vi "HFP Generator.vi"() -> ()   [LabVIEW 2015]
doc: "Example VI that demonstrates all library features."
uses:
  PL HFP Generator.lvclass
panel:
  in  "series":u16(ring) items=["Plasma G20", "Plasma GK"]
  in  "read configuration":bool
  out "measurements":T1 {"SWR timer state" items=["off"=0, "counting"=2, "counting and skipping"=3, "protection"=4]; "rf power"."Ppump, W" items=["500", "1000", "2000", "3000", "4000", "6000", "8000"]; "power ramp state" items=["off", "ramp up", "full power", "ramp down", "off, awaiting reset"]}
  in  "configuration":T2={"power on"=FALSE, "rf on"=FALSE, "control mode"=0, "disable rf"=FALSE, "power"={"Pfwd, W"=50, "Pload, W"=50, "Pmax, W"=1000, "ramp"={"mode"=0, "up time, s"=0, "down time, s"=0}}, "modulation"={"mode"=0, "f, Hz"=1000, "pulse time, s"=1.0, "duty cycle, %"=50.0, "Ppause, W"=50}, "SWR timer"={"on"=FALSE, "Pthreshold, W"=0, "count time, s"=0, "skip time, s"=0}, "phase"={"phase, °"=0.0, "mode"=1}} {"phase"."mode" items=["slave", "master"]; "modulation"."mode" items=["off"=0, "internal full"=2, "internal partial"=3, "external full"=4, "external partial"=5]; "power"."ramp"."mode" items=["off", "ramp up", "ramp up and down", "ramp down"]; "control mode" items=["Pload", "Pfwd"]}
  out "device information":T3
  in  "stop bits":u16(ring)=10 items=["1.0"=10, "2.0"=20]
  in  "parity":enum16{"None", "Odd", "Even", "Mark", "Space"}(ring)
  out "HFP Gen":refnum<class "PL HFP Generator.lvclass">
  in  "port":refnum<visa-resource-name>
  in  "address":u8=1
  in  "baud rate":u32(ring)=19200 items=["9600"=9600, "19200"=19200, "38400"=38400]
  out "error":errorcluster
  in  "stop":bool
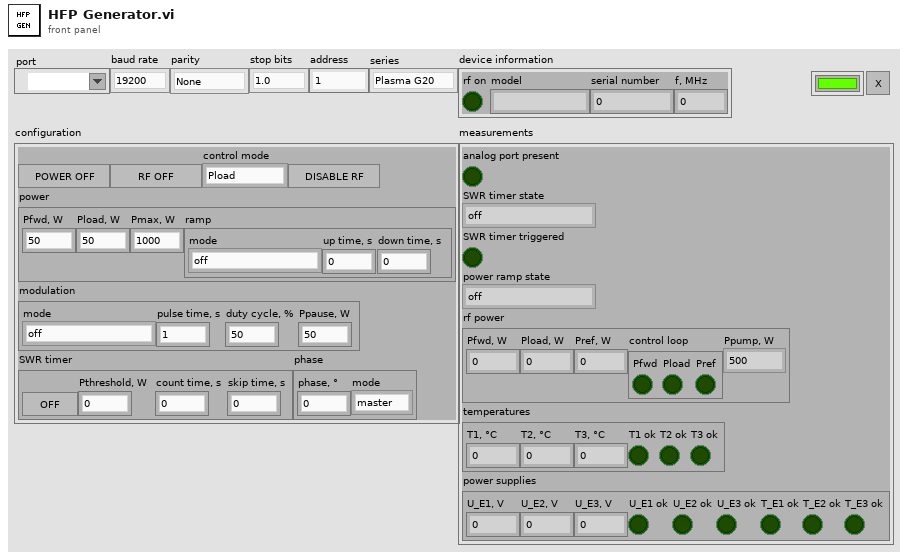
[diagram p1: front panel]
types:
  T1 = cluster{"analog port present":bool, "SWR timer state":u8, "SWR timer triggered":bool, "power ramp state":u8, "rf power":cluster{"Pfwd, W":dbl, "Pload, W":dbl, "Pref, W":dbl, "control loop":cluster{"Pfwd":bool, "Pload":bool, "Pref":bool}, "Ppump, W":u8}, "temperatures":cluster{"T1, °C":dbl, "T2, °C":dbl, "T3, °C":dbl, "T1 ok":bool, "T2 ok":bool, "T3 ok":bool}, "power supplies":cluster{"U_E1, V":dbl, "U_E2, V":dbl, "U_E3, V":dbl, "U_E1 ok":bool, "U_E2 ok":bool, "U_E3 ok":bool, "T_E1 ok":bool, "T_E2 ok":bool, "T_E3 ok":bool}}
  T2 = cluster{"power on":bool, "rf on":bool, "control mode":u8, "disable rf":bool, "power":cluster{"Pfwd, W":u16, "Pload, W":u16, "Pmax, W":u16, "ramp":cluster{"mode":u8, "up time, s":u8, "down time, s":u8}}, "modulation":cluster{"mode":u8, "f, Hz":u16, "pulse time, s":dbl, "duty cycle, %":dbl, "Ppause, W":u16}, "SWR timer":cluster{"on":bool, "Pthreshold, W":u8, "count time, s":u8, "skip time, s":u8}, "phase":cluster{"phase, °":dbl, "mode":u8}}
  T3 = cluster{"rf on":bool, "model":string, "serial number":u16, "f, MHz":dbl}
  T4 = cluster{"power on":bool, "rf on":bool, "control mode":u8, "modulation mode":u8, "SWR timer on":bool, "power ramp mode":u8}
  T5 = cluster{"power on":bool, "rf on":bool, "control mode":u8, "mode":u8, "on":bool, "disable rf":bool}
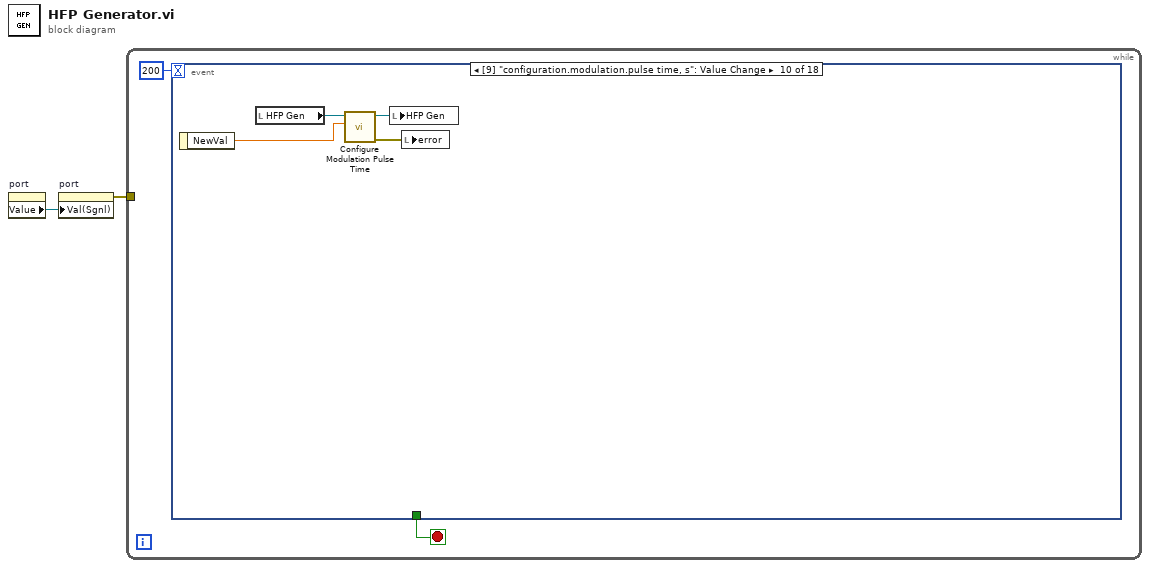
[diagram p0: block diagram]
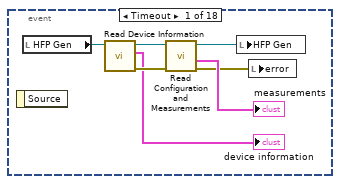
[diagram p2: hidden frame]
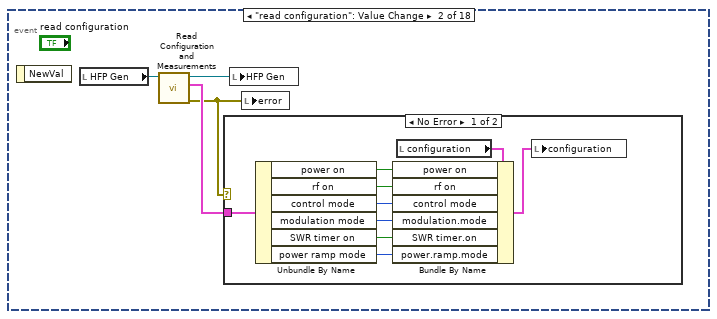
[diagram p3: hidden frame]
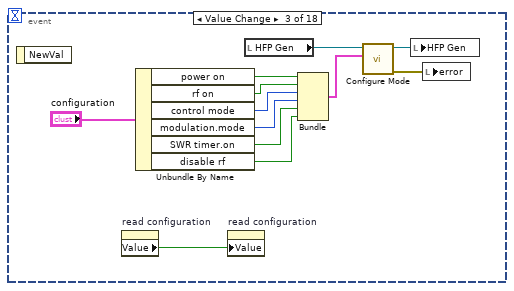
[diagram p5: hidden frame]
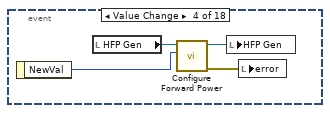
[diagram p6: hidden frame]
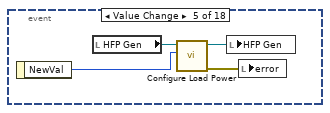
[diagram p7: hidden frame]
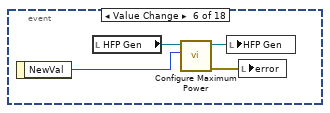
[diagram p8: hidden frame]
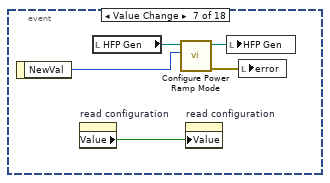
[diagram p9: hidden frame]
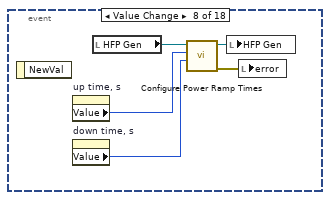
[diagram p10: hidden frame]
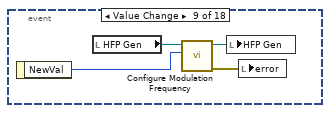
[diagram p11: hidden frame]
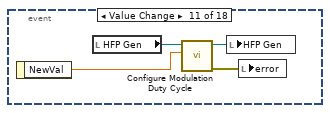
[diagram p12: hidden frame]
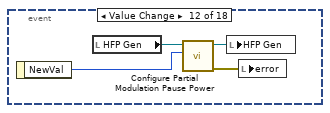
[diagram p13: hidden frame]
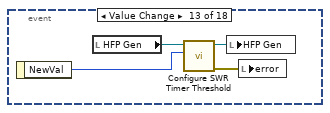
[diagram p14: hidden frame]
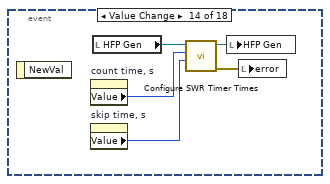
[diagram p15: hidden frame]
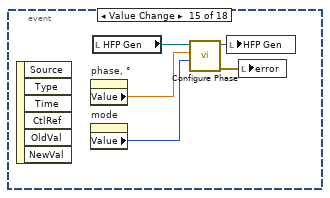
[diagram p16: hidden frame]
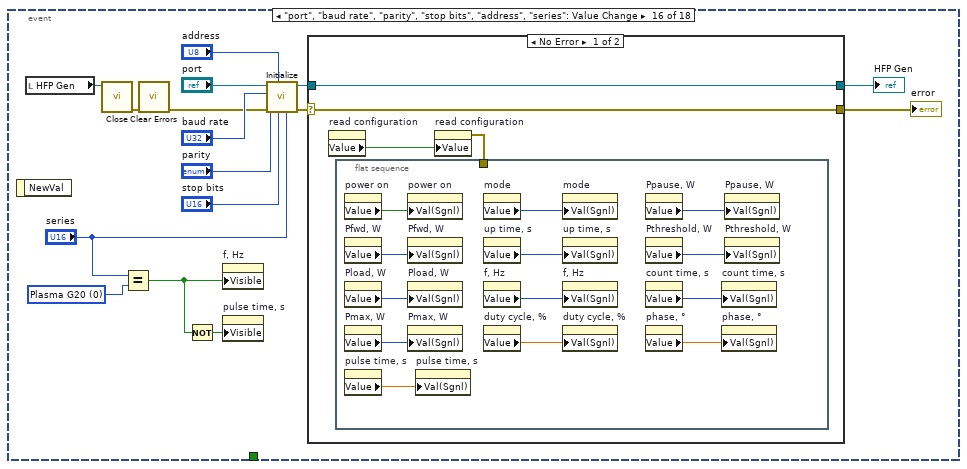
[diagram p17: hidden frame]
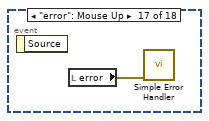
[diagram p19: hidden frame]
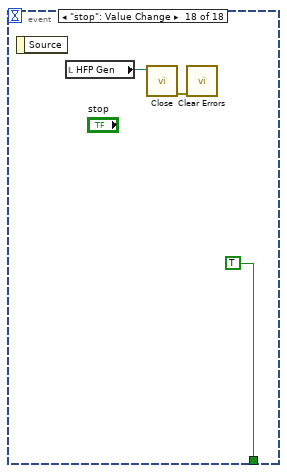
[diagram p20: hidden frame]
diagram:
  n1 = property on="port" class="VISAName"() -> ("Value"=w1:refnum<visa-resource-name>)  [unwired: 2 in, 2 out]
  n2 = property on="port" class="VISAName"("Val(Sgnl)"=w1) -> (error out=w2:errorcluster)  [unwired: 2 in, 1 out]
  n3 = while {
    tunnel: w2 -> [_]
    stop <- w3 stop-if-true
    n4 = event shown="[9] \"configuration.modulation.pulse time, s\": Value Change" {
      selector: _ -> [_ _ _ _ _ _ _ _ _ _ _ _ _ _ _ _ _ _]
      dyn-events: _ -> [_ _ _ _ _ _ _ _ _ _ _ _ _ _ _ _ _ _]
      timeout: 200 -> [_ _ _ _ _ _ _ _ _ _ _ _ _ _ _ _ _ _]
      tunnel: [_ _ _ _ _ _ _ _ _ _ _ _ _ _ _ _ _ TRUE ("stop")] -> w3
      event Timeout {
        n5 = event-data() -> ()  [unwired: 1 in, 1 out]
        n6 = local read "HFP Gen"() -> (w11:refnum<class "PL HFP Generator.lvclass">)
        n7 = call "Read Device Information.vi"("HFP Gen in"=w11) -> ("error out"=w8:errorcluster, "information"=→"device information":T3, "HFP Gen out"=w10:refnum<class "PL HFP Generator.lvclass">)  [unwired: 8 in]
        n8 = call "Read Configuration and Measurements.vi"("error in (no error)"=w8, "HFP Gen in"=w10) -> ("error out"=w5:errorcluster, "measurements"=→"measurements":T1, "HFP Gen out"=w9:refnum<class "PL HFP Generator.lvclass">)  [unwired: 6 in, 1 out]
        n9 = local write "HFP Gen"(w9) -> ()
        n10 = local write "error"(w5) -> ()
      }
      event "read configuration": Value Change {
        n11 = event-data() -> ()  [unwired: 1 in, 1 out]
        n12 = local read "HFP Gen"() -> (w15:refnum<class "PL HFP Generator.lvclass">)
        n13 = call "Read Configuration and Measurements.vi"("HFP Gen in"=w15) -> ("error out"=w12:errorcluster, "configuration"=w13:T4, "HFP Gen out"=w14:refnum<class "PL HFP Generator.lvclass">)  [unwired: 7 in, 1 out]
        n14 = case shown="No Error" w12 {
          tunnel: w13 -> [w24 _]
          frame No Error {
            n15 = Unbundle By Name(w24) -> ("power on"=w22:bool, "rf on"=w21:bool, "control mode"=w20:u8, "modulation mode"=w19:u8, "SWR timer on"=w18:bool, "power ramp mode"=w17:u8)
            n16 = local read "configuration"() -> (w16:T2)
            n17 = Bundle By Name(cluster=w16, "power on"=w22, "rf on"=w21, "control mode"=w20, "modulation.mode"=w19, "SWR timer.on"=w18, "power.ramp.mode"=w17) -> (w23:T2)
            n18 = local write "configuration"(w23) -> ()
          }
          frame Error {
          }
        }
        n19 = local write "HFP Gen"(w14) -> ()
        n20 = local write "error"(w12) -> ()
      }
      event "configuration.power on", "configuration.rf on", "configuration.control mode", "configuration.modulation.mode", "configuration.SWR timer.on", "configuration.disable rf": Value Change {
        n21 = event-data() -> ()  [unwired: 1 in, 1 out]
        n22 = property on="read configuration" class="Bool (strict)"() -> ("Value"=w25:bool)  [unwired: 2 in, 2 out]
        n23 = Unbundle By Name("configuration") -> ("power on"=w32:bool, "rf on"=w31:bool, "control mode"=w30:u8, "modulation.mode"=w29:u8, "SWR timer.on"=w28:bool, "disable rf"=w27:bool)
        n24 = property on="read configuration" class="Bool (strict)"("Value"=w25) -> ()  [unwired: 2 in, 2 out]
        n25 = local read "HFP Gen"() -> (w34:refnum<class "PL HFP Generator.lvclass">)
        n26 = Bundle("power on"=w32, "rf on"=w31, "control mode"=w30, "mode"=w29, "on"=w28, "disable rf"=w27) -> (w26:T5)  [unwired: 1 in]
        n27 = call "Configure Mode.vi"("mode"=w26, "HFP Gen in"=w34) -> ("error out"=w36:errorcluster, "HFP Gen out"=w35:refnum<class "PL HFP Generator.lvclass">)  [unwired: 8 in]
        n28 = local write "HFP Gen"(w35) -> ()
        n29 = local write "error"(w36) -> ()
      }
      event "configuration.power.Pfwd, W": Value Change {
        n30 = event-data() -> ("NewVal"=w37:u16)  [unwired: 1 in]
        n31 = local read "HFP Gen"() -> (w40:refnum<class "PL HFP Generator.lvclass">)
        n32 = call "Configure Forward Power.vi"("Pfwd, W"=w37, "HFP Gen in"=w40) -> ("error out"=w38:errorcluster, "HFP Gen out"=w39:refnum<class "PL HFP Generator.lvclass">)  [unwired: 8 in]
        n33 = local write "HFP Gen"(w39) -> ()
        n34 = local write "error"(w38) -> ()
      }
      event "configuration.power.Pload, W": Value Change {
        n35 = event-data() -> ("NewVal"=w41:u16)  [unwired: 1 in]
        n36 = local read "HFP Gen"() -> (w43:refnum<class "PL HFP Generator.lvclass">)
        n37 = call "Configure Load Power.vi"("Pload, W"=w41, "HFP Gen in"=w43) -> ("error out"=w42:errorcluster, "HFP Gen out"=w44:refnum<class "PL HFP Generator.lvclass">)  [unwired: 8 in]
        n38 = local write "HFP Gen"(w44) -> ()
        n39 = local write "error"(w42) -> ()
      }
      event "configuration.power.Pmax, W": Value Change {
        n40 = event-data() -> ("NewVal"=w45:u16)  [unwired: 1 in]
        n41 = local read "HFP Gen"() -> (w46:refnum<class "PL HFP Generator.lvclass">)
        n42 = call "Configure Maximum Power.vi"("Pmax, W"=w45, "HFP Gen in"=w46) -> ("error out"=w47:errorcluster, "HFP Gen out"=w48:refnum<class "PL HFP Generator.lvclass">)  [unwired: 8 in]
        n43 = local write "HFP Gen"(w48) -> ()
        n44 = local write "error"(w47) -> ()
      }
      event "configuration.power.ramp.mode": Value Change {
        n45 = event-data() -> ("NewVal"=w50:u8)  [unwired: 1 in]
        n46 = property on="read configuration" class="Bool (strict)"() -> ("Value"=w49:bool)  [unwired: 2 in, 2 out]
        n47 = local read "HFP Gen"() -> (w51:refnum<class "PL HFP Generator.lvclass">)
        n48 = call "Configure Power Ramp Mode.vi"("power ramp mode"=w50, "HFP Gen in"=w51) -> ("error out"=w52:errorcluster, "HFP Gen out"=w53:refnum<class "PL HFP Generator.lvclass">)  [unwired: 8 in]
        n49 = property on="read configuration" class="Bool (strict)"("Value"=w49) -> ()  [unwired: 2 in, 2 out]
        n50 = local write "HFP Gen"(w53) -> ()
        n51 = local write "error"(w52) -> ()
      }
      event "configuration.power.ramp.up time, s", "configuration.power.ramp.down time, s": Value Change {
        n52 = event-data() -> ()  [unwired: 1 in, 1 out]
        n53 = property on="up time, s" class="DigNum (strict)"() -> ("Value"=w55:u8)  [unwired: 2 in, 2 out]
        n54 = property on="down time, s" class="DigNum (strict)"() -> ("Value"=w54:u8)  [unwired: 2 in, 2 out]
        n55 = local read "HFP Gen"() -> (w56:refnum<class "PL HFP Generator.lvclass">)
        n56 = call "Configure Power Ramp Times.vi"("ramp-down time, s"=w54, "ramp-up time, s"=w55, "HFP Gen in"=w56) -> ("error out"=w57:errorcluster, "HFP Gen out"=w58:refnum<class "PL HFP Generator.lvclass">)  [unwired: 7 in]
        n57 = local write "HFP Gen"(w58) -> ()
        n58 = local write "error"(w57) -> ()
      }
      event "configuration.modulation.f, Hz": Value Change {
        n59 = event-data() -> ("NewVal"=w59:u16)  [unwired: 1 in]
        n60 = local read "HFP Gen"() -> (w61:refnum<class "PL HFP Generator.lvclass">)
        n61 = call "Configure Modulation Frequency.vi"("f, Hz"=w59, "HFP Gen in"=w61) -> ("error out"=w60:errorcluster, "HFP Gen out"=w62:refnum<class "PL HFP Generator.lvclass">)  [unwired: 8 in]
        n62 = local write "HFP Gen"(w62) -> ()
        n63 = local write "error"(w60) -> ()
      }
      event "configuration.modulation.pulse time, s": Value Change {
        n64 = event-data() -> ("NewVal"=w63:dbl)  [unwired: 1 in]
        n65 = local read "HFP Gen"() -> (w65:refnum<class "PL HFP Generator.lvclass">)
        n66 = call "Configure Modulation Pulse Time.vi"("pulse time, s"=w63, "HFP Gen in"=w65) -> ("error out"=w64:errorcluster, "HFP Gen out"=w66:refnum<class "PL HFP Generator.lvclass">)  [unwired: 8 in]
        n67 = local write "HFP Gen"(w66) -> ()
        n68 = local write "error"(w64) -> ()
      }
      event "configuration.modulation.duty cycle, %": Value Change {
        n69 = event-data() -> ("NewVal"=w67:dbl)  [unwired: 1 in]
        n70 = local read "HFP Gen"() -> (w68:refnum<class "PL HFP Generator.lvclass">)
        n71 = call "Configure Modulation Duty Cycle.vi"("duty cycle, %"=w67, "HFP Gen in"=w68) -> ("error out"=w69:errorcluster, "HFP Gen out"=w70:refnum<class "PL HFP Generator.lvclass">)  [unwired: 8 in]
        n72 = local write "HFP Gen"(w70) -> ()
        n73 = local write "error"(w69) -> ()
      }
      event "configuration.modulation.Ppause, W": Value Change {
        n74 = event-data() -> ("NewVal"=w71:u16)  [unwired: 1 in]
        n75 = local read "HFP Gen"() -> (w72:refnum<class "PL HFP Generator.lvclass">)
        n76 = call "Configure Partial Modulation Pause Power.vi"("Ppause, W"=w71, "HFP Gen in"=w72) -> ("error out"=w73:errorcluster, "HFP Gen out"=w74:refnum<class "PL HFP Generator.lvclass">)  [unwired: 8 in]
        n77 = local write "HFP Gen"(w74) -> ()
        n78 = local write "error"(w73) -> ()
      }
      event "configuration.SWR timer.Pthreshold, W": Value Change {
        n79 = event-data() -> ("NewVal"=w75:u8)  [unwired: 1 in]
        n80 = local read "HFP Gen"() -> (w76:refnum<class "PL HFP Generator.lvclass">)
        n81 = call "Configure SWR Timer Threshold.vi"("Pthreshold, W"=w75, "HFP Gen in"=w76) -> ("error out"=w77:errorcluster, "HFP Gen out"=w78:refnum<class "PL HFP Generator.lvclass">)  [unwired: 8 in]
        n82 = local write "HFP Gen"(w78) -> ()
        n83 = local write "error"(w77) -> ()
      }
      event "configuration.SWR timer.count time, s", "configuration.SWR timer.skip time, s": Value Change {
        n84 = event-data() -> ()  [unwired: 1 in, 1 out]
        n85 = property on="count time, s" class="DigNum (strict)"() -> ("Value"=w80:u8)  [unwired: 2 in, 2 out]
        n86 = property on="skip time, s" class="DigNum (strict)"() -> ("Value"=w79:u8)  [unwired: 2 in, 2 out]
        n87 = local read "HFP Gen"() -> (w83:refnum<class "PL HFP Generator.lvclass">)
        n88 = call "Configure SWR Timer Times.vi"("skip time, s"=w79, "count time, s"=w80, "HFP Gen in"=w83) -> ("error out"=w81:errorcluster, "HFP Gen out"=w82:refnum<class "PL HFP Generator.lvclass">)  [unwired: 7 in]
        n89 = local write "HFP Gen"(w82) -> ()
        n90 = local write "error"(w81) -> ()
      }
      event "configuration.phase.phase, °", "configuration.phase.mode": Value Change {
        n91 = event-data() -> ()  [unwired: 1 in, 6 out]
        n92 = property on="phase, °" class="DigNum (strict)"() -> ("Value"=w85:dbl)  [unwired: 2 in, 2 out]
        n93 = property on="mode" class="Ring (strict)"() -> ("Value"=w84:u8)  [unwired: 2 in, 2 out]
        n94 = local read "HFP Gen"() -> (w88:refnum<class "PL HFP Generator.lvclass">)
        n95 = call "Configure Phase.vi"("mode"=w84, "phase, °"=w85, "HFP Gen in"=w88) -> ("error out"=w86:errorcluster, "HFP Gen out"=w87:refnum<class "PL HFP Generator.lvclass">)  [unwired: 7 in]
        n96 = local write "HFP Gen"(w87) -> ()
        n97 = local write "error"(w86) -> ()
      }
      event "port", "baud rate", "parity", "stop bits", "address", "series": Value Change {
        w91 = u16 0 items=["Plasma G20", "Plasma GK"]
        n98 = event-data() -> ()  [unwired: 1 in, 1 out]
        n99 = local read "HFP Gen"() -> (w102:refnum<class "PL HFP Generator.lvclass">)
        n100 = call-dynamic "Close.vi"("HFP Gen in"=w102) -> ("error out"=w101:errorcluster)  [unwired: 10 in]
        n101 = Equal?(x="series", y=w91) -> (x = y?=w90:bool)
        n102 = call <vilib>:"Clear Errors.vi"("error in (no error)"=w101) -> ("error out"=w100:errorcluster)  [unwired: 5 in, 1 out]
        n103 = Not(x=w90) -> (.not. x?=w89:bool)
        n104 = property on="f, Hz" class="DigNum (strict)"("Visible"=w90) -> ()  [unwired: 2 in, 2 out]
        n105 = property on="pulse time, s" class="DigNum (strict)"("Visible"=w89) -> ()  [unwired: 2 in, 2 out]
        n106 = call "Initialize.vi"("series (Plasma G20)"="series", "stop bits (1.0)"="stop bits", "address (1)"="address", "error in (no error)"=w100, "parity (none)"="parity", "baud rate (19200)"="baud rate", "port"="port") -> ("error out"=w96:errorcluster, "HFP Gen out"=w94:refnum<class "PL HFP Generator.lvclass">)  [unwired: 3 in]
        n107 = case shown="No Error" w96 {
          selector: w96 -> [w107 w123]
          tunnel: [w107 w123] -> w95
          tunnel: w94 -> [w108 w122]
          tunnel: [w108 w122] -> w93
          frame No Error {
            n108 = property on="read configuration" class="Bool (strict)"() -> ("Value"=w106:bool)  [unwired: 2 in, 2 out]
            n109 = flat-sequence {
              tunnel: w105 -> [_]
              frame #0 {
                n110 = property on="power on" class="Bool (strict)"() -> ("Value"=w121:bool)  [unwired: 2 in, 2 out]
                n111 = property on="Pfwd, W" class="DigNum (strict)"() -> ("Value"=w120:u16)  [unwired: 2 in, 2 out]
                n112 = property on="Pload, W" class="DigNum (strict)"() -> ("Value"=w119:u16)  [unwired: 2 in, 2 out]
                n113 = property on="Pmax, W" class="DigNum (strict)"() -> ("Value"=w118:u16)  [unwired: 2 in, 2 out]
                n114 = property on="pulse time, s" class="DigNum (strict)"() -> ("Value"=w109:dbl)  [unwired: 2 in, 2 out]
                n115 = property on="power on" class="Bool (strict)"("Val(Sgnl)"=w121) -> ()  [unwired: 2 in, 2 out]
                n116 = property on="Pfwd, W" class="DigNum (strict)"("Val(Sgnl)"=w120) -> ()  [unwired: 2 in, 2 out]
                n117 = property on="Pload, W" class="DigNum (strict)"("Val(Sgnl)"=w119) -> ()  [unwired: 2 in, 2 out]
                n118 = property on="Pmax, W" class="DigNum (strict)"("Val(Sgnl)"=w118) -> ()  [unwired: 2 in, 2 out]
                n119 = property on="pulse time, s" class="DigNum (strict)"("Val(Sgnl)"=w109) -> ()  [unwired: 2 in, 2 out]
                n120 = property on="mode" class="Ring (strict)"() -> ("Value"=w114:u8)  [unwired: 2 in, 2 out]
                n121 = property on="up time, s" class="DigNum (strict)"() -> ("Value"=w115:u8)  [unwired: 2 in, 2 out]
                n122 = property on="f, Hz" class="DigNum (strict)"() -> ("Value"=w116:u16)  [unwired: 2 in, 2 out]
                n123 = property on="duty cycle, %" class="DigNum (strict)"() -> ("Value"=w117:dbl)  [unwired: 2 in, 2 out]
                n124 = property on="mode" class="Ring (strict)"("Val(Sgnl)"=w114) -> ()  [unwired: 2 in, 2 out]
                n125 = property on="up time, s" class="DigNum (strict)"("Val(Sgnl)"=w115) -> ()  [unwired: 2 in, 2 out]
                n126 = property on="f, Hz" class="DigNum (strict)"("Val(Sgnl)"=w116) -> ()  [unwired: 2 in, 2 out]
                n127 = property on="duty cycle, %" class="DigNum (strict)"("Val(Sgnl)"=w117) -> ()  [unwired: 2 in, 2 out]
                n128 = property on="Ppause, W" class="DigNum (strict)"() -> ("Value"=w113:u16)  [unwired: 2 in, 2 out]
                n129 = property on="Pthreshold, W" class="DigNum (strict)"() -> ("Value"=w112:u8)  [unwired: 2 in, 2 out]
                n130 = property on="count time, s" class="DigNum (strict)"() -> ("Value"=w111:u8)  [unwired: 2 in, 2 out]
                n131 = property on="phase, °" class="DigNum (strict)"() -> ("Value"=w110:dbl)  [unwired: 2 in, 2 out]
                n132 = property on="count time, s" class="DigNum (strict)"("Val(Sgnl)"=w111) -> ()  [unwired: 2 in, 2 out]
                n133 = property on="phase, °" class="DigNum (strict)"("Val(Sgnl)"=w110) -> ()  [unwired: 2 in, 2 out]
                n134 = property on="Ppause, W" class="DigNum (strict)"("Val(Sgnl)"=w113) -> ()  [unwired: 2 in, 2 out]
                n135 = property on="Pthreshold, W" class="DigNum (strict)"("Val(Sgnl)"=w112) -> ()  [unwired: 2 in, 2 out]
              }
            }
            n136 = property on="read configuration" class="Bool (strict)"("Value"=w106) -> (error out=w105:errorcluster)  [unwired: 2 in, 1 out]
          }
          frame Error {
          }
        }
        "error" <- w95
        "HFP Gen" <- w93
      }
      event "error": Mouse Up {
        n137 = event-data() -> ()  [unwired: 1 in, 1 out]
        n138 = local read "error"() -> (w124:errorcluster)
        n139 = call <vilib>:"Simple Error Handler.vi"("error in (no error)"=w124) -> ()  [unwired: 4 in, 5 out]
      }
      event "stop": Value Change {
        n140 = event-data() -> ()  [unwired: 1 in, 1 out]
        n141 = local read "HFP Gen"() -> (w125:refnum<class "PL HFP Generator.lvclass">)
        n142 = call-dynamic "Close.vi"("HFP Gen in"=w125) -> ("error out"=w126:errorcluster)  [unwired: 10 in]
        n143 = call <vilib>:"Clear Errors.vi"("error in (no error)"=w126) -> ()  [unwired: 5 in, 2 out]
      }
    }
  }
